vi "ReadResistanceSim921.vi"(9 "Port":i32, 10 "GPIB":refnum<visa-resource-name>) -> (2 "Resistance":dbl, 3 "GPIB":refnum<visa-resource-name>)   [LabVIEW 2019]
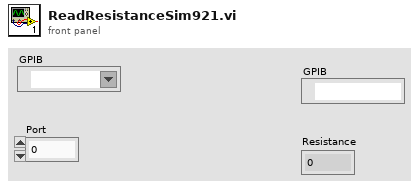
[diagram p1: front panel]
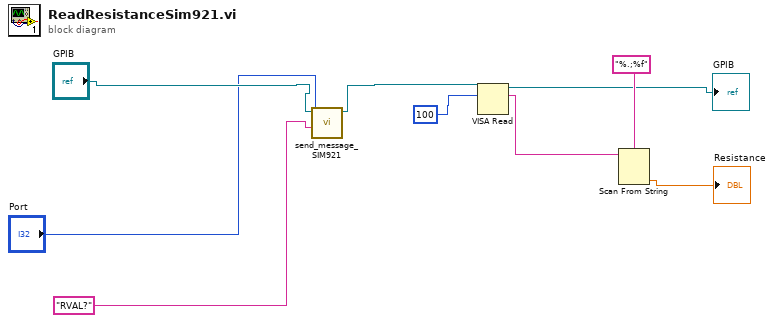
[diagram p0: block diagram]
diagram:
  n1 = call "send_message_SIM921.vi"("Message (\"\")"="RVAL?", "Channel (0: SIM900)"="Port", "VISA resource name"="GPIB") -> ("VISA resource name out"=w4:refnum<visa-resource-name>)  [unwired: 7 in, 1 out]
  n2 = VISA Read(VISA resource name=w4, byte count=100) -> (VISA resource name out=→"GPIB":refnum<visa-resource-name>, read buffer=w8:string)  [unwired: 1 in, 2 out]
  n3 = Scan From String(format string="%.;%f", input string=w8) -> (output 1=→"Resistance":dbl)  [unwired: 3 in, 3 out]
